vi "Test Section Cluster Tools.vi"() -> ()   [LabVIEW 2017]
uses:
  fb7ec740-fa34-4e2e-931b-2d8ee0f6284f.vi
  31061775-ad27-4825-bed1-ddc8a47e55d7.vi
  JSON text to Variant (path).vi
  Find Item.vi
  String Subset.vi
  JSON text to Variant.vi
  <vilib>/Utility/Data Type/Get Type Information.vi
  Parsing/Parse Full Path or Item Name.vi
  Offset/Find Item Locations by Path.vi
  JSONtext.lvlib
panel:
  out "Rest of Input String":string
  out "data 2":T1
  out "<JSON> 2":string caption="<JSON>Sections"
  out "data":cluster{"3124":i32, "efqwf":string}
  out "error out":errorcluster
  out "<JSON>":string
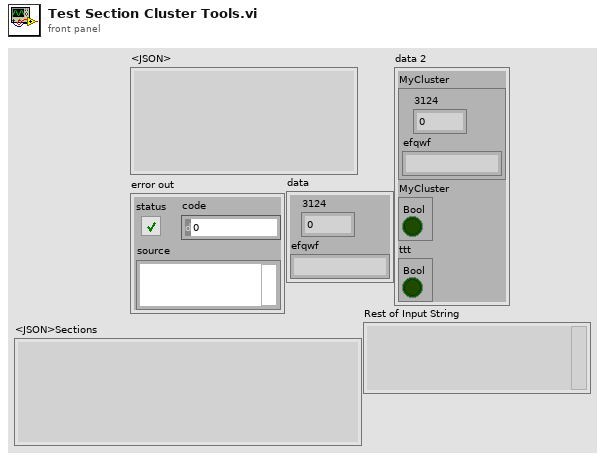
[diagram p1: front panel]
types:
  T1 = cluster{"MyCluster":cluster{"3124":i32, "efqwf":string}, "MyCluster":cluster{"Bool":bool}, "ttt":cluster{"Bool":bool}}
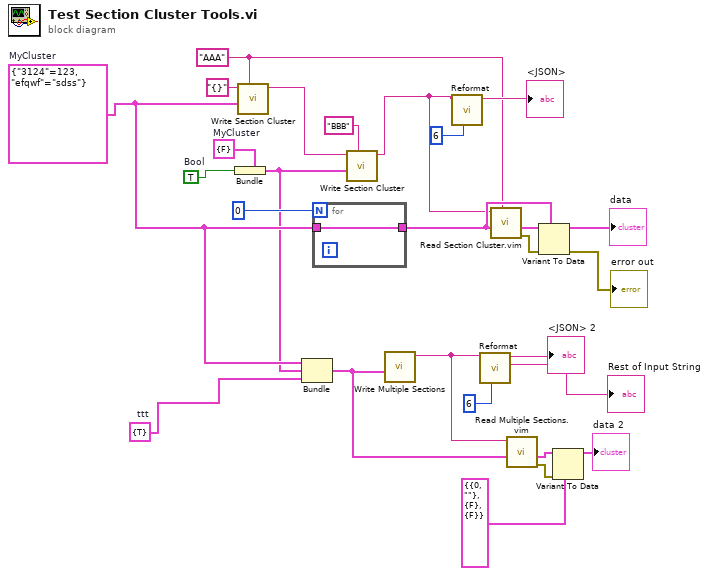
[diagram p0: block diagram]
diagram:
  w1 = "AAA" ("Section Name (Cluster Name)")
  w14 = cluster{"Bool":bool} {"Bool"=TRUE}  # ttt
  w19 = cluster{"Bool":bool} {"Bool"=FALSE}  # MyCluster
  w25 = TRUE  # Bool
  w16 = cluster{"3124":i32, "efqwf":string} {"3124"=123, "efqwf"="sdss"}  # MyCluster
  n1 = Bundle(cluster=w19, "Bool"=w25) -> (w15:cluster{"Bool":bool})
  n2 = call "Write Section Cluster.vi"("Section Name (Cluster Name)"=w1, "Section Cluster"=w16, "JSON Sections"="{}" ("JSON Object to merge into")) -> ("<JSON>"=w26:string)  [unwired: 6 in, 1 out]
  n3 = Bundle("MyCluster"=w16, "MyCluster"=w15, "ttt"=w14) -> (w10:T1)  [unwired: 1 in]
  n4 = for {
    N: 0 -> [_]
    tunnel: [w28] -> w20
    tunnel: w16 -> [w28]
  }
  n5 = call "Write Section Cluster.vi"("Section Name (Cluster Name)"="BBB" ("Path into Object"), "Section Cluster"=w15, "JSON Sections"=w26) -> ("<JSON>"=w6:string)  [unwired: 6 in, 1 out]
  n6 = call "Write Multiple Sections.vi"("Section Cluster"=w10) -> ("<JSON>"=w13:string)  [unwired: 8 in, 1 out]
  n7 = call "Reformat.vi"("Pretty Print Levels"=6, "JSON"=w6) -> ("<JSON>First JSON Value\n\n<JSON>"=→"<JSON>":string)  [unwired: 6 in, 3 out]
  n8 = call "Reformat.vi"("Pretty Print Levels"=6, "JSON"=w13) -> ("Rest of Input String"=→"Rest of Input String":string, "<JSON>First JSON Value\n\n<JSON>"=→"<JSON> 2":string)  [unwired: 6 in, 2 out]
  n9 = call "Read Section Cluster.vim"("Section (Cluster Name)"=w1, "Section Cluster"=w20, "JSON Sections"=w6) -> ("error out"=w22:errorcluster, "Cluster set from section"=w23:cluster{"3124":i32, "efqwf":string})  [unwired: 5 in, 1 out]
  n10 = call "Read Multiple Sections.vim"("Cluster of Section Clusters"=w10, "JSON Sections"=w13) -> ("error out"=w12:errorcluster, "Cluster out"=w11:T1)  [unwired: 7 in]
  n11 = Variant To Data(error in=w22, type=w20, Variant=w23) -> (data=→"data":cluster{"3124":i32, "efqwf":string}, error out=→"error out":errorcluster)
  n12 = Variant To Data(error in=w12, type=T1 {"MyCluster"={"3124"=0, "efqwf"=""}, "MyCluster"={"Bool"=FALSE}, "ttt"={"Bool"=FALSE}} ("output cluster"), Variant=w11) -> (data=→"data 2":T1)  [unwired: 1 out]
